vi "experiment state global.vi"() -> ()   [LabVIEW 2013]
panel:
  out "data directory and name":T1={"data directory"=path "B:/lady gaga/olfaction/EtAc Spatial Linear 0 to 50 ppm 20 cm 10min_habituation/CS/20130105/1650", "file stub"="CS_EtAc_SLi_0to50_20_10min_habituation_201301051650"}
  in  "experiment phase":T2
  out "experiment state":T3
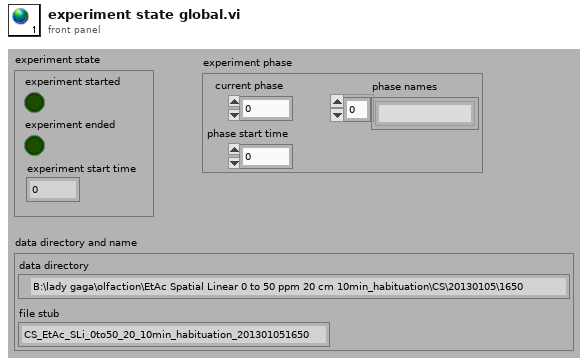
[diagram p1: front panel]
types:
  T1 = cluster{"data directory":path, "file stub":string}
  T2 = cluster{"current phase":u16, "phase start time":dbl, "phase names":string[]}
  T3 = cluster{"experiment started":bool, "experiment ended":bool, "experiment start time":u32}
diagram:
